vi "Debug.vi"(11 "Compiled":T1 {"Nodes"."Monitor"."Network"."Name" format="%.0x"; "Nodes"."Sim"."Network"."Name" format="%.0x"; "XNET"."Termination" items=["Off", "On"]}) -> (3 "output cluster":T1 {"Nodes"."Monitor"."Network"."Name" format="%.0x"; "Nodes"."Sim"."Network"."Name" format="%.0x"; "XNET"."Termination" items=["Off", "On"]})   [LabVIEW 2015, in "J1939 Addon System Explorer.lvlib"]
uses:
  J1939 Addon System Explorer.lvlib
  Shared/Types/Compile Addon Settings.ctl
  Shared/Types/XNET Settings.ctl
  Shared/Types/SysDef FPGA Settings.ctl
  Shared/Types/Compiled.Node Settings.ctl
  Shared/Types/Compiled Monitor Tool Settings.ctl
  Shared/Types/Monitor Settings.ctl
  Shared/Types/Device Settings.ctl
  Shared/Types/Incoming Settings.ctl
  Shared/Types/Incoming Frame Settings.ctl
  <vilib>/NI Veristand/Custom Device API/Block Data Reference.ctl
  <vilib>/NI Veristand/Custom Device API/Data Reference.ctl
  Shared/Types/Outgoing Settings.ctl
  Shared/Types/Outgoing Frame Settings.ctl
  Shared/Types/Outgoing Event Trigger Types.ctl
  Shared/Types/Exported Frame Settings.ctl
  Shared/Types/Exported Frame Type.ctl
  Shared/Types/Exported Protection Settings.ctl
  Shared/Types/Protection Type.ctl
  Shared/Types/InputChannelConfiguration.ctl
  Shared/Types/Exported Counter Settings.ctl
  Shared/Types/Complied Simulated Device Settings.ctl
  Shared/Types/Compiled Simulated Settings.ctl
  Shared/J1939 Addon Shared.lvlib
  <vilib>/NI VeriStand/Custom Device API/Custom Device API.lvlib
panel:
  in  "Exit":bool
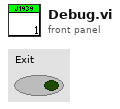
[diagram p1: front panel]
types:
  T1 = typedef "J1939 Addon Shared.lvlib/Compile Addon Settings.ctl" = cluster{"XNET":T2, "Bitfile":T3, "Nodes":T4, "Name":string}
  T2 = typedef "J1939 Addon Shared.lvlib/XNET Settings.ctl" = cluster{"Database":refnum<k21>, "Cluster":refnum<k21>, "Port":string, "Baud rate [Bd]":u32, "Termination":u32, "Incoming Decimation":u32, "Outgoing Decimation":u32}
  T3 = typedef "J1939 Addon Shared.lvlib/SysDef FPGA Settings.ctl" = cluster{"RT Path":path, "RIO Device":string, "Enable":bool}
  T4 = typedef "J1939 Addon Shared.lvlib/Compiled.Node Settings.ctl" = cluster{"Monitor":T5, "Sim":T21[]}
  T5 = typedef "J1939 Addon Shared.lvlib/Compiled Monitor Tool Settings.ctl" = cluster{"Network":T6, "Data":T7}
  T6 = typedef "J1939 Addon Shared.lvlib/Monitor Settings.ctl" = cluster{"Address":u8, "Name":u64, "Include DA":bool}
  T7 = typedef "J1939 Addon Shared.lvlib/Device Settings.ctl" = cluster{"Incoming":T8, "Outgoing":T12}
  T8 = typedef "J1939 Addon Shared.lvlib/Incoming Settings.ctl" = cluster{"Signals":string[], "Frames":T9[], "Data.Refs":T10[], "Data.Values":dbl[], "Timing.Use":bool, "Timing.Refs":T10[], "Timing.Values":dbl[], "Timing.Index":i32[]}
  T9 = typedef "J1939 Addon Shared.lvlib/Incoming Frame Settings.ctl" = cluster{"Signals":string[], "PGN":u32}
  T10 = typedef "Custom Device API.lvlib/Block Data Reference.ctl" = cluster{"Data Reference":T11, "Offset":u64, "Length":u64}
  T11 = typedef "Custom Device API.lvlib/Data Reference.ctl" = i32
  T12 = typedef "J1939 Addon Shared.lvlib/Outgoing Settings.ctl" = cluster{"Frames":T13[], "Data.Refs":T10[], "Data.Values":dbl[], "Disable.Refs":T10[], "Disable.Values":dbl[], "Trigger.Refs":T10[], "Trigger.Values":dbl[], "Frames.CountersAndProtections":T15[]}
  T13 = typedef "J1939 Addon Shared.lvlib/Outgoing Frame Settings.ctl" = cluster{"Signals":string[], "Channel Array Position":cluster{"Offset":u32, "Length":u32}, "PGN":u32, "Cyclic?":bool, "Disable?":bool, "Disable.Index":i32, "Trigger":T14, "Trigger.Index":i32}
  T14 = typedef "J1939 Addon Shared.lvlib/Outgoing Event Trigger Types.ctl" = enum16{"Channel value change", "Trigger channel (not zero)", "Channel value change or trigger channel (not zero)", "Trigger channel (any value change)", "Channel value change or trigger channel (any value change)"}
  T15 = typedef "J1939 Addon Shared.lvlib/Exported Frame Settings.ctl" = cluster{"Type":T16, "Frame ID":u32, "Payload Length":u32, "Signal XNET Paths":string[], "Frame.PrevData":dbl[], "VS Offset":i32, "VS Length":i32, "Generation Period":u32, "Has Protection?":bool, "Protection Configurations":T17[], "Has Counter":bool, "Counter Configurations":T20[], "Has Disable?":bool, "Disable VS Index":i32, "Transmit Trigger":T14, "Trigger VS Index":i32}
  T16 = typedef "J1939 Addon Shared.lvlib/Exported Frame Type.ctl" = enum16{"Periodic", "Event", "Periodic/Event"}
  T17 = typedef "J1939 Addon Shared.lvlib/Exported Protection Settings.ctl" = cluster{"Protection Frame Index":i32, "Protection Type":T18, "Data Indeces":i32[], "Initialized Data Array":dbl[], "Protection Signal XNET Paths":string[], "CRC Channels":T19[], "Protection VS Update Index":i32}
  T18 = typedef "J1939 Addon Shared.lvlib/Protection Type.ctl" = enum16{"Arb ID + Bytes Checksum with Inversion", "Arb ID + Bytes CRC with Inversion", "Reversed Raw Signal Checksum with Inversion"}
  T19 = typedef "J1939 Addon Shared.lvlib/InputChannelConfiguration.ctl" = cluster{"Start Bit":i32, "Name":string, "Number of bits":i32, "Scale":dbl, "Offset":dbl, "Data Type":u32}
  T20 = typedef "J1939 Addon Shared.lvlib/Exported Counter Settings.ctl" = cluster{"Counter Frame Index":i32, "Max Count":dbl, "Counter VS Index":i32}
  T21 = typedef "J1939 Addon Shared.lvlib/Complied Simulated Device Settings.ctl" = cluster{"Network":T6, "Data":T7, "DTCs":T22}
  T22 = typedef "J1939 Addon Shared.lvlib/Compiled Simulated Settings.ctl" = cluster{"DM1.Ref":T10[], "DM1.Value":dbl[], "DM1.Enable.Ref":T10[], "DM1.Enable.Value":dbl[], "DM2.Ref":T10[], "DM2.Value":dbl[], "DM2.Enable.Ref":T10[], "DM2.Enable.Value":dbl[]}
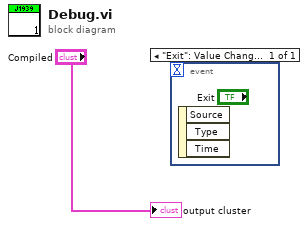
[diagram p0: block diagram]
diagram:
  n1 = event shown="[0] \"Exit\": Value Change" {
    selector: _ -> [_]
    dyn-events: _ -> [_]
    timeout: _ -> [_]
    event "Exit": Value Change {
      n2 = event-data() -> ()  [unwired: 1 in, 3 out]
    }
  }
  "output cluster" <- "Compiled"
